vi "0037-Sub_calc_Si7021.vi"(8 "humi":u8[](array[numeric]), 10 "temp":u8[](array[numeric])) -> (1 "humi":dbl, 3 "temp":dbl)   [LabVIEW 2014]
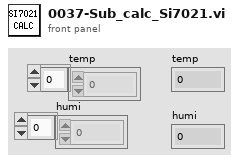
[diagram p1: front panel]
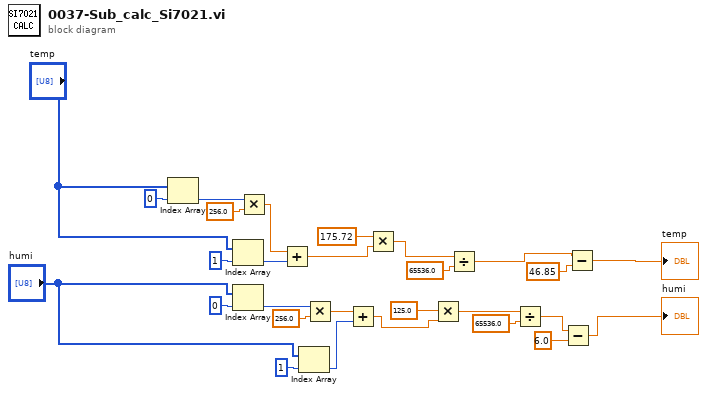
[diagram p0: block diagram]
diagram:
  n1 = Index Array(array="temp", index=0 ("指標")) -> (element=w16:u8)
  n2 = Index Array(array="temp", index=1 ("指標")) -> (element=w19:u8)
  n3 = Index Array(array="humi", index=0 ("指標")) -> (element=w26:u8)
  n4 = Multiply(x=w16, y=256.0) -> (x*y=w18:dbl)
  n5 = Add(x=w18, y=w19) -> (x+y=w7:dbl)
  n6 = Index Array(array="humi", index=1 ("指標")) -> (element=w27:u8)
  n7 = Multiply(x=w26, y=256.0) -> (x*y=w24:dbl)
  n8 = Add(x=w24, y=w27) -> (x+y=w2:dbl)
  n9 = Multiply(x=175.72, y=w7) -> (x*y=w6:dbl)
  n10 = Multiply(x=125.0, y=w2) -> (x*y=w1:dbl)
  n11 = Divide(x=w6, y=65536.0) -> (x/y=w4:dbl)
  n12 = Divide(x=w1, y=65536.0) -> (x/y=w10:dbl)
  n13 = Subtract(x=w10, y=6.0) -> (x-y=→"humi":dbl)
  n14 = Subtract(x=w4, y=46.85 ("x")) -> (x-y=→"temp":dbl)
